vi "Projeto_Final.vi"() -> ()   [LabVIEW 2021]
uses:
  <vilib>/Instr/_visa.llb/VISA Configure Serial Port (Instr).vi
panel:
  out "Tempo Inicial":u32
  out "D":dbl
  out "remaining string":string
  out "error out 6":errorcluster={"status"=FALSE, "code"=1073676418, "source"="VISA Close in projeto v5.vi"}
  out "String enviada para o Arduino":string="27  0  0  0  -10"
  out "error out 5":errorcluster={"status"=TRUE, "code"=-1073807346, "source"="VISA Read in projeto v5.vi"}
  out "error out 4":errorcluster={"status"=TRUE, "code"=-1073807346, "source"="VISA Write in projeto v5.vi"}
  out "error out 3":errorcluster
  out "error out 2":errorcluster
  out "error out":errorcluster={"status"=TRUE, "code"=1, "source"="Scan From String (arg 1) in projeto v5.vi"}
  out "Tempo Decorrido (s)":dbl=0.9981727600097656 caption="Elapsed Time (s)"
  in  "Pressione para \ncriar um ficheiro de texto":bool
  out "PV":dbl=-9.968760743918754
  in  "Insira o file path antes \nde iniciar o programa":path=path "C:/Users/Ana Pereira/Desktop/sac.txt"
  out "Control Action (CA)":dbl
  out "I":dbl
  out "P":dbl
  out "Set Point":dbl
  out "?":cluster{"Set Point":dbl, "Process Value":dbl}(graph)={"Set Point"=-9.968760743918754, "Process Value"=0.0}
  in  "Disturbance(DIS)":dbl(slide)=11.616161616161616 scale=10.0..20.0
  in  "D":dbl
  in  "I":dbl
  in  "P":dbl
  in  "Set Point":dbl(slide)=26.666666666666664 scale=0.0..100.0
  in  "VISA resource name":refnum<visa-resource-name>="COM3"
  out "Resposta do Arduino":string
  in  "Stop":bool
  # "Controlo de uma Planta Industrial a partir de um algoritmo PID desenvolvido em Arduino\n2021/2022 - Sensores, Atuadores e Controlo - Projeto\nAna Beatriz Vitorino Pereira (up201905457) \nEma Beatriz Salgado Fernandes (up201909527) \nMariana Sampaio Terroso (up202103314)"
  # "Ligação Arduino- Labview"
  # "Exportação de dados"
  # "Erros"
  # "Input"
  # "Output"
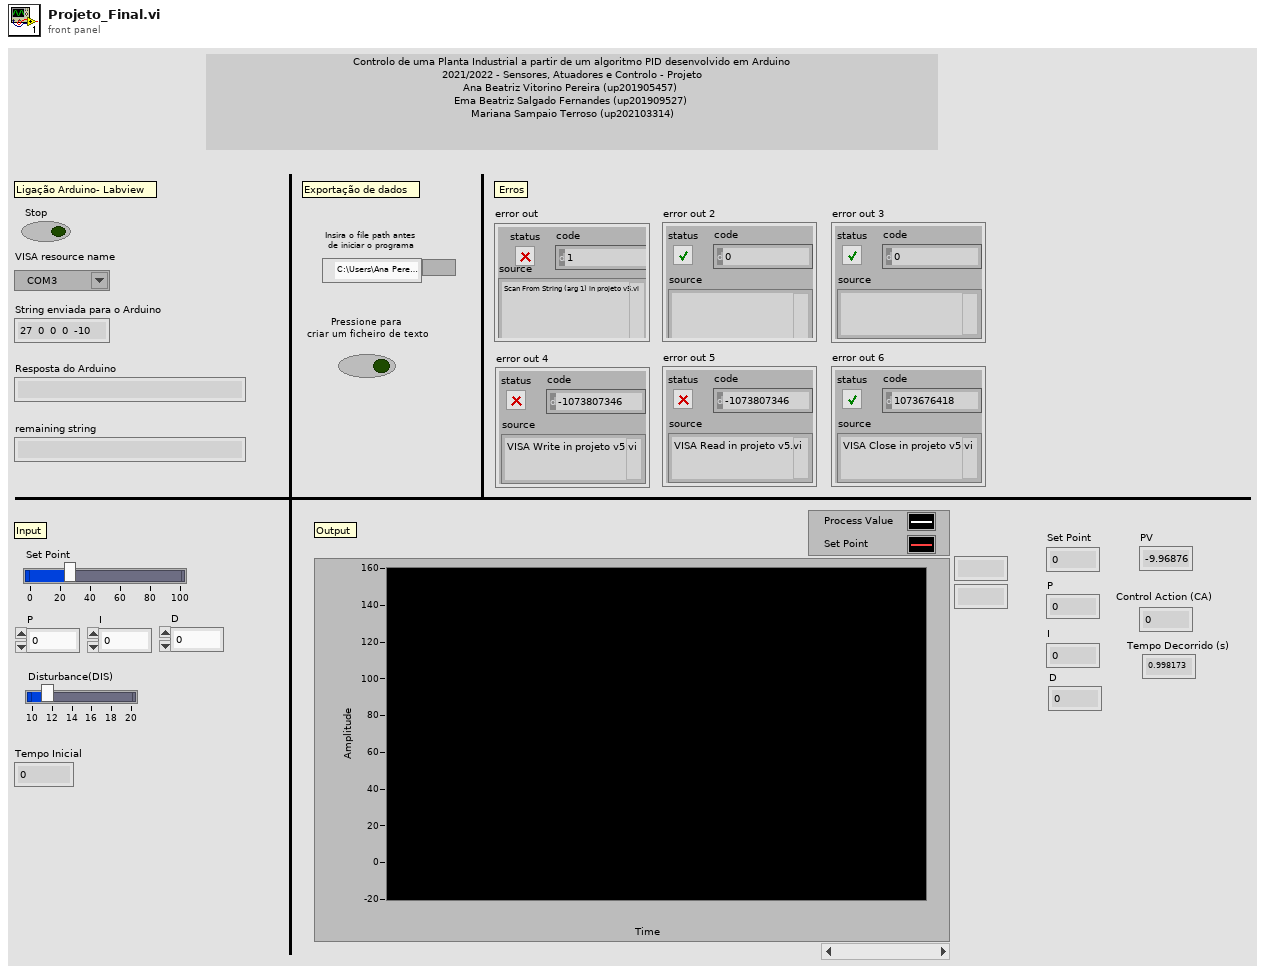
[diagram p1: front panel]
types:
  T1 = enum16{"open", "replace", "create", "open or create", "replace or create", "replace or create with confirmation"}
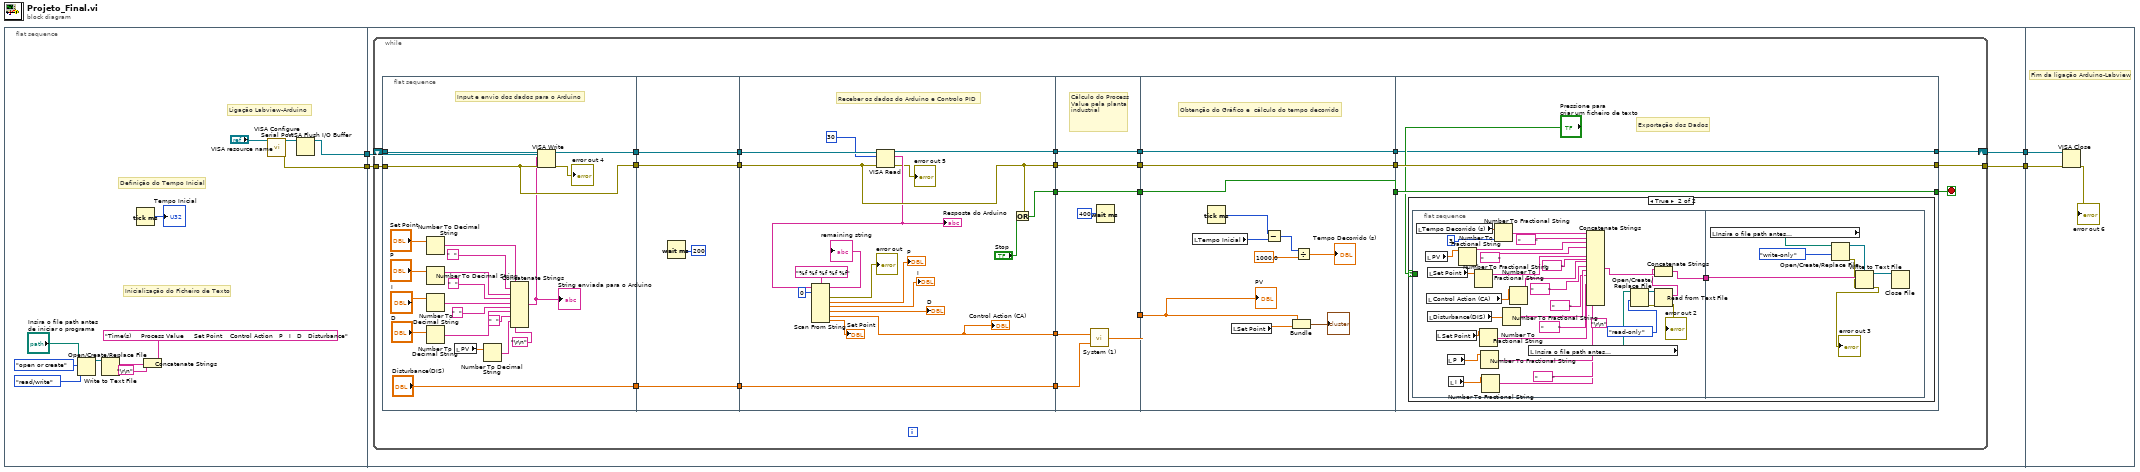
[diagram p0: block diagram]
diagram:
  n1 = flat-sequence {
    tunnel: [w8] -> w4
    tunnel: [w6] -> w1
    tunnel: w4 -> [w20]
    tunnel: [w19] -> w3
    tunnel: [w18] -> w2
    tunnel: w1 -> [w17]
    tunnel: w3 -> [w153]
    tunnel: w2 -> [w152]
    frame #0 {
      # "Definição do Tempo Inicial"
      # "Inicialização do Ficheiro de Texto"
      # "Ligação Labview-Arduino"
      n2 = Open/Create/Replace File(file path (use dialog)="Insira o file path antes \nde iniciar o programa", operation (0:open)=T1."open or create", access (0:read/write)=enum16{"read/write", "read-only", "write-only"}."read/write") -> (refnum out=w14:refnum<file>)  [unwired: 3 in, 2 out]
      n3 = Tick Count (ms)() -> (millisecond timer value=→"Tempo Inicial":u32)
      n4 = Concatenate Strings("Time(s)     Process Value     Set Point    Control Action   P   I   D   Disturbance", "\r\n") -> (w9:string)
      n5 = Write to Text File(file (use dialog)=w14, text=w9) -> ()  [unwired: 2 in, 3 out]
      n6 = call-poly "VISA Configure Serial Port"("VISA resource name"="VISA resource name") -> ("VISA resource name out"=w7:refnum<visa-resource-name>, "error out"=w8:errorcluster)  [unwired: 13 in]
      n7 = VISA Flush I/O Buffer(VISA resource name=w7) -> (VISA resource name out=w6:refnum<visa-resource-name>)  [unwired: 2 in, 1 out]
    }
    frame #1 {
      n8 = while {
        tunnel: [w42] -> w19
        shift-right: [w43] -> w18
        shift-left: w17 -> [w41]
        tunnel: w20 -> [w39]
        stop <- w40 stop-if-true
        n9 = flat-sequence {
          tunnel: w41 -> [w64]
          tunnel: [w63] -> w35
          tunnel: [w62] -> w33
          tunnel: ["Disturbance(DIS)"] -> w31
          tunnel: w39 -> [w62]
          tunnel: w35 -> [w68]
          tunnel: [w68] -> w34
          tunnel: w33 -> [w67]
          tunnel: [w67] -> w32
          tunnel: w31 -> [w66]
          tunnel: [w66] -> w30
          tunnel: [w85] -> w29
          tunnel: [w84] -> w28
          tunnel: [w83] -> w27
          tunnel: w34 -> [w77]
          tunnel: w32 -> [w83]
          tunnel: w30 -> [w80]
          tunnel: [w80] -> w26
          tunnel: [w72] -> w25
          tunnel: w29 -> [w93]
          tunnel: [w93] -> w24
          tunnel: w28 -> [w92]
          tunnel: [w92] -> w23
          tunnel: w27 -> [w91]
          tunnel: [w91] -> w22
          tunnel: [w88] -> w21
          tunnel: w26 -> [w90]
          tunnel: w25 -> [w89]
          tunnel: [w104] -> w38
          tunnel: [w103] -> w37
          tunnel: [w102] -> w36
          tunnel: w21 -> [w95]
          tunnel: w22 -> [w102]
          tunnel: w23 -> [w103]
          tunnel: w24 -> [w104]
          tunnel: [w107] -> w42
          tunnel: [w105] -> w43
          tunnel: [w108] -> w40
          tunnel: w38 -> [w108]
          tunnel: w37 -> [w105]
          tunnel: w36 -> [w107]
          frame #0 {
            # "Input e envio dos dados para o Arduino"
            n10 = Number To Decimal String(number="Set Point") -> (decimal integer string=w59:string)  [unwired: 1 in]
            n11 = Number To Decimal String(number="D") -> (decimal integer string=w49:string)  [unwired: 1 in]
            n12 = Number To Decimal String(number="P") -> (decimal integer string=w53:string)  [unwired: 1 in]
            n13 = Number To Decimal String(number="I") -> (decimal integer string=w51:string)  [unwired: 1 in]
            n14 = local read "PV"() -> (w45:dbl)
            n15 = Number To Decimal String(number=w45) -> (decimal integer string=w47:string)  [unwired: 1 in]
            n16 = Concatenate Strings(w59, "  " ("string"), w53, "  " ("string"), w51, "  " ("string"), w49, "  " ("string"), w47, "\r\n") -> (w58:string)
            "String enviada para o Arduino" <- w58
            n17 = VISA Write(VISA resource name=w64, write buffer=w58, error in (no error)=w62) -> (VISA resource name out=w63:refnum<visa-resource-name>, error out=→"error out 4":errorcluster)  [unwired: 1 out]
          }
          frame #1 {
            n18 = Wait (ms)(milliseconds to wait=u32 200) -> ()  [unwired: 1 out]
          }
          frame #2 {
            # "Receber os dados do Arduino e Controlo PID"
            n19 = VISA Read(VISA resource name=w77, byte count=u32 30, error in (no error)=w83) -> (VISA resource name out=w84:refnum<visa-resource-name>, read buffer=w82:string, error out=→"error out 5":errorcluster)  [unwired: 1 out]
            "Resposta do Arduino" <- w82
            n20 = Scan From String(format string="%f %f %f %f %f", input string=w82, initial scan location=u32 0) -> (remaining string=→"remaining string":string, error out=→"error out":errorcluster, output 1=→"P":dbl, output 2=→"I":dbl, output 3=→"D":dbl, output 4=w72:dbl, output 5=→"Set Point":dbl)  [unwired: 6 in, 1 out]
            "Control Action (CA)" <- w72
            n21 = Or(x=w83, y="Stop") -> (x .or. y?=w85:bool)
          }
          frame #3 {
            # "Cálculo do Process Value pela planta industrial"
            n22 = call "System (1).vi"("Disturbance"=w90, "Control Action"=w89) -> ("Process Value"=w88:dbl)
            n23 = Wait (ms)(milliseconds to wait=u32 400) -> ()  [unwired: 1 out]
          }
          frame #4 {
            # "Obtenção do Gráfico e  cálculo do tempo decorrido"
            n24 = local read "Tempo Inicial"() -> (w100:u32)
            n25 = Tick Count (ms)() -> (millisecond timer value=w99:u32)
            n26 = local read "Set Point"() -> (w101:dbl)
            n27 = Subtract(x=w99, y=w100) -> (x-y=w96:u32)
            n28 = Bundle("Process Value"=w95, "Set Point"=w101) -> (→"?":cluster{"Process Value":dbl, "Set Point":dbl})  [unwired: 1 in]
            n29 = Divide(x=w96, y=1000.0) -> (x/y=→"Tempo Decorrido (s)":dbl)
            "PV" <- w95
          }
          frame #5 {
            # "Exportação dos Dados"
            n30 = case shown="True" "Pressione para \ncriar um ficheiro de texto" {
              selector: "Pressione para \ncriar um ficheiro de texto" -> [_ w109]
              frame False {
              }
              frame True {
                n31 = flat-sequence {
                  tunnel: [w135] -> w110
                  tunnel: w109 -> [_]
                  tunnel: w110 -> [w150]
                  frame #0 {
                    n32 = local read "Tempo Decorrido (s)"() -> (w113:dbl)
                    n33 = local read "PV"() -> (w114:dbl)
                    n34 = local read "Control Action (CA)"() -> (w129:dbl)
                    n35 = local read "Set Point"() -> (w132:dbl)
                    n36 = local read "Disturbance(DIS)"() -> (w126:dbl)
                    n37 = local read "Set Point"() -> (w123:dbl)
                    n38 = local read "P"() -> (w122:dbl)
                    n39 = local read "I"() -> (w121:dbl)
                    n40 = Number To Fractional String(number=w114) -> (F-format string=w141:string)  [unwired: 3 in]
                    n41 = Number To Fractional String(number=w132) -> (F-format string=w131:string)  [unwired: 3 in]
                    n42 = Number To Fractional String(number=w123) -> (F-format string=w120:string)  [unwired: 3 in]
                    n43 = Number To Fractional String(number=w122) -> (F-format string=w118:string)  [unwired: 3 in]
                    n44 = Number To Fractional String(number=w121) -> (F-format string=w116:string)  [unwired: 3 in]
                    n45 = Number To Fractional String(number=w113, precision (6)=i16 3) -> (F-format string=w143:string)  [unwired: 2 in]
                    n46 = Number To Fractional String(number=w126) -> (F-format string=w125:string)  [unwired: 3 in]
                    n47 = Number To Fractional String(number=w129) -> (F-format string=w128:string)  [unwired: 3 in]
                    n48 = local read "Insira o file path antes \nde iniciar o programa"() -> (w133:path)
                    n49 = Concatenate Strings(w143, "       ", w141, "       ", w131, "       ", w128, "       ", w125, "       ", w120, "       ", w118, "       ", w116, "\r\n") -> (w139:string)
                    n50 = Open/Create/Replace File(file path (use dialog)=w133, access (0:read/write)=enum16{"read/write", "read-only", "write-only"}."read-only") -> (refnum out=w137:refnum<file>, error out=w112:errorcluster)  [unwired: 4 in, 1 out]
                    n51 = Read from Text File(file (use dialog)=w137, error in=w112) -> (text=w136:string, error out=→"error out 2":errorcluster)  [unwired: 2 in, 2 out]
                    n52 = Concatenate Strings(w136, w139) -> (w135:string)
                  }
                  frame #1 {
                    n53 = local read "Insira o file path antes \nde iniciar o programa"() -> (w149:path)
                    n54 = Open/Create/Replace File(file path (use dialog)=w149, access (0:read/write)=enum16{"read/write", "read-only", "write-only"}."write-only") -> (refnum out=w147:refnum<file>, error out=w145:errorcluster)  [unwired: 4 in, 1 out]
                    n55 = Write to Text File(file (use dialog)=w147, text=w150, error in=w145) -> (refnum out=w146:refnum<file>, error out=→"error out 3":errorcluster)  [unwired: 1 in, 1 out]
                    n56 = Close File(refnum=w146) -> ()  [unwired: 1 in, 2 out]
                  }
                }
              }
            }
          }
        }
      }
    }
    frame #2 {
      # "Fim da ligação Arduino-Labview"
      n57 = VISA Close(VISA resource name=w152, error in (no error)=w153) -> (error out=→"error out 6":errorcluster)
    }
  }
